vi "Global Log Handling Capability Example.vi"() -> ()   [LabVIEW 2017, in "Global Log Handling Capability Example.lvlib"]
doc: "### Global Log Handling Capability(Global Log Handling Capability Example.vi)\n\n#### Overview\n\nDemonstrates global log handling capability of CSM. This example calls 30 sub-modules that continuously generate events. The main VI captures these events and uses the Global Log APIs to calculate and display key processing metrics, such as LogInQ, changing speed, and handling speed.\n\nUse this example to benchmark global log performance of CSM and as a reference for custom implementations.\n\n#### Introduction\n\nThis example demonstrates global log handling capability of CSM. This example calls 30 sub-modules that continuously generate events. The main VI captures these events and uses the Global Log APIs to calculate and display key processing metrics, such as LogInQ, changing speed, and handling speed.\n\nUse this example to benchmark global log performance of CSM and as a reference for custom implementations.\n\n#### Steps\n\nStep 1: Asynchronously call 30 CSM submodules, each of which will then generate events continuously.\n\nStep 2: Starts the CSM Watchdog thread to ensure that all asynchronously started CSM modules exit properly after the main program exits.\n\nStep 3: Use CSM's built-in global log APIs to capture and calculate some typical logging capability figures.\n\nStep 4: Exit the caller and all the other running CSM modules."
uses:
  Global Log Handling Capability Example.lvlib
  user.lib/_NEVSTOP/Communicable State Machine(CSM)/Utility/_support/Periodic String Filter Level.ctl
  user.lib/_NEVSTOP/Communicable State Machine(CSM)/Utility/Periodic String Filter Setting.ctl
  user.lib/_NEVSTOP/Communicable State Machine(CSM)/Communicable State Machine.lvlib
  user.lib/_NEVSTOP/Communicable State Machine(CSM)/addons/Watchdog/CSM Watchdog.lvlib
  user.lib/_NEVSTOP/Communicable State Machine(CSM)/_Shared/CSM Shared.lvlib
panel:
  out "size(s)":i32
  in  "Module Num":i32=30
  out "log handling Speed(#/s)":dbl(graph)
  out "Since Exiting(s)":dbl format="%.2f"
  out "LogInQ":i32
  out "State History":string
  out "log handling Speed(#/s)":dbl
  out "LogInQ changing Speed(#/s)":dbl
  out "Level":T1
  out "Module Names":string[](array[string])
  in  "Exit Modules":bool
  # "Set before run VI"
  # "#CSM-Example Overview\n\nDemonstrates invoking a CSM submodule in a side loop. Externally, this module interacts like a standard CSM submodule, but note its specific API and status change behavior."
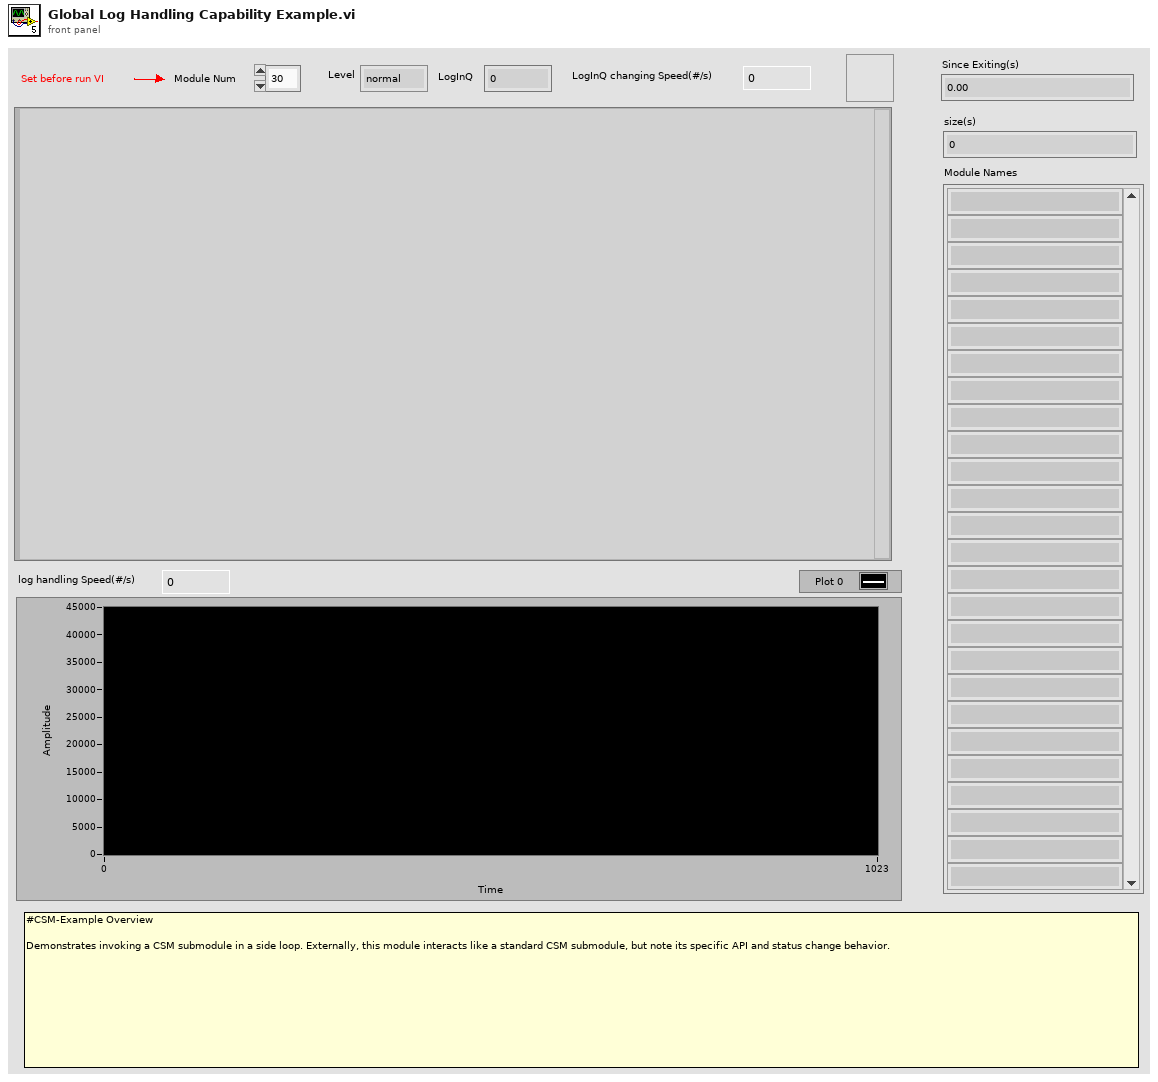
[diagram p1: front panel]
types:
  T1 = typedef "Communicable State Machine.lvlib/Periodic String Filter Level.ctl" = enum16{"normal", "L1", "L2", "L3", "L4"}
  T2 = typedef "Communicable State Machine.lvlib/Periodic String Filter Setting.ctl" = cluster{"threashold(#/s)":dbl, "Check Peroid(s)":dbl}
  T3 = typedef "Communicable State Machine.lvlib/_CSM_GlobalLog_MSG.ctl" = cluster{"Name (\"\" to Use UUID)":string, "Current State":string, "Arguments":string, "Source Message":T4, "Source Module":string, "Complete(T)/Start(F)":bool, "LogType":T5, "Time Stamp":timestamp}
  T4 = typedef "Communicable State Machine.lvlib/_CSM_Response Source Message.ctl" = cluster{"‘State":string, "’Arguments":string, "’Error":errorcluster}
  T5 = typedef "Communicable State Machine.lvlib/_CSM_GlobalLog_MSG_TYPE.ctl" = enum16{"User Log", "State Change", "Status", "Interrupt", "Register", "Unregister", "Error Log", "Module Created", "Module Destroyed"}
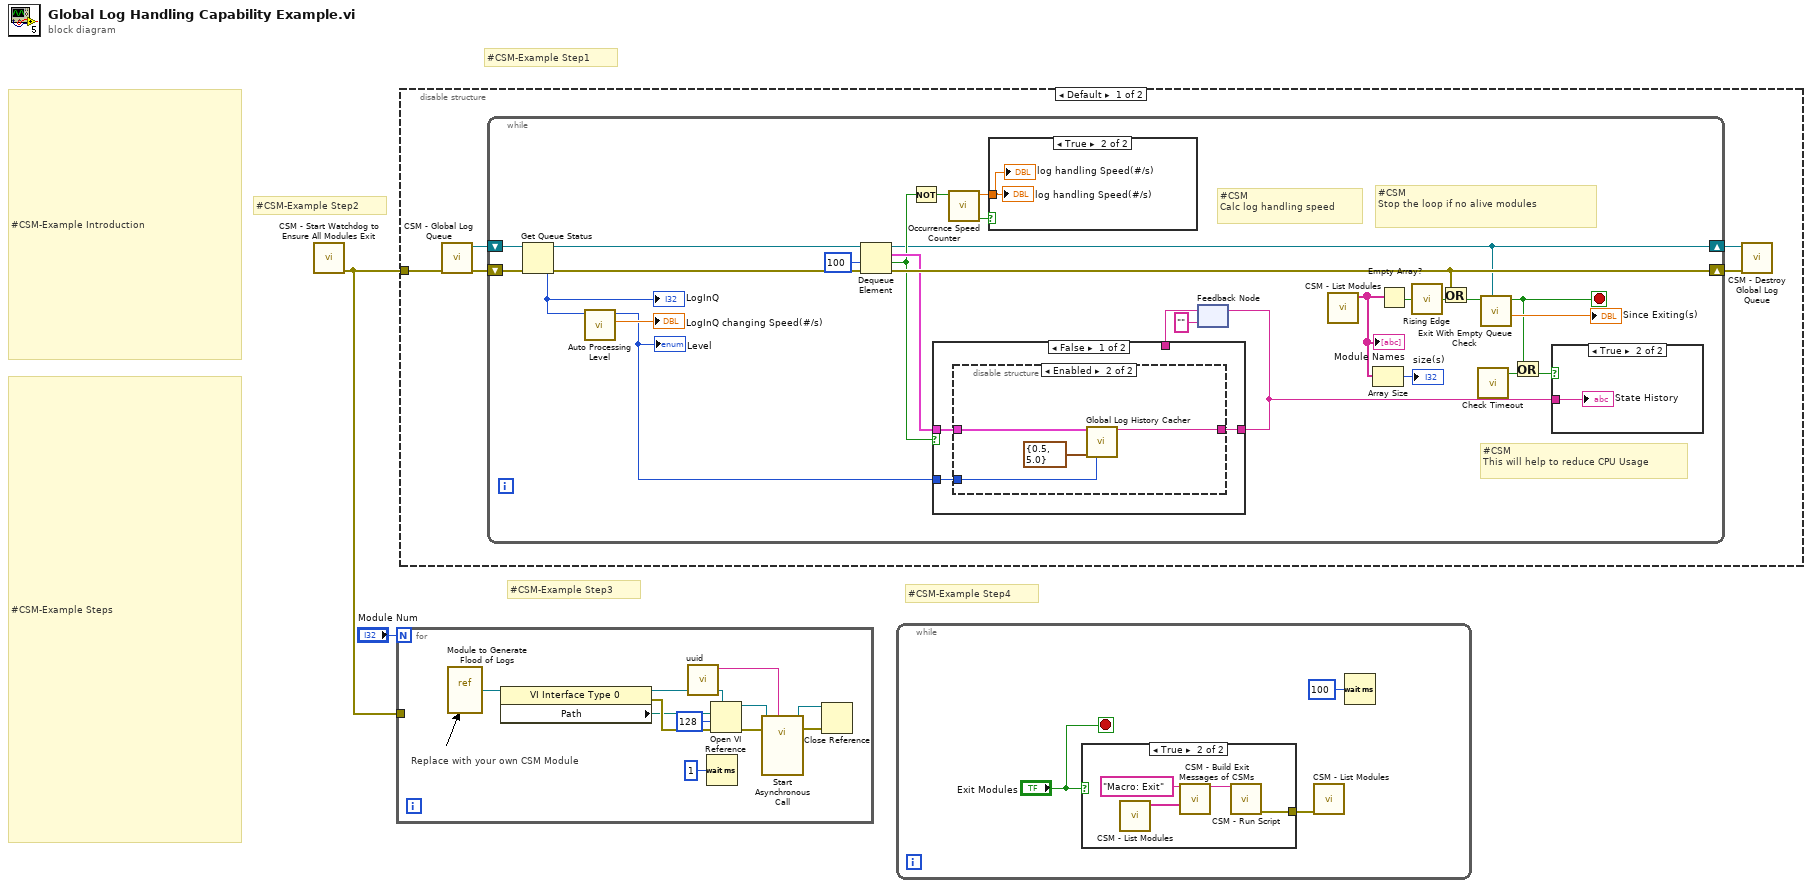
[diagram p0: block diagram]
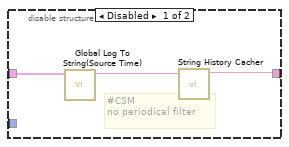
[diagram p3: hidden frame]
diagram:
  # "#CSM-Example Step4"
  # "#CSM-Example Step3"
  # "#CSM-Example Step2"
  # "#CSM-Example Step1"
  # "#CSM-Example Steps"
  # "#CSM-Example Introduction"
  n1 = call "CSM - Start Watchdog to Ensure All Modules Exit.vi"() -> ("error out"=w1:errorcluster)  [unwired: 11 in]
  n2 = for {
    N: "Module Num" -> [_]
    tunnel: w1 -> [_]
    # "Replace with your own CSM Module"
    n3 = vi-ref "Module to Generate Flood of Logs.vi"() -> (w6:refnum<vi>)
    n4 = property class="VI Interface Type 0"(reference=w6) -> (reference out=w10:refnum<vi>, error out=w8:errorcluster, "Path"=w7:path)  [unwired: 1 in]
    n5 = call "uuid.vi"() -> ("UUID"=w4:string)  [unwired: 11 in]
    n6 = Wait (ms)(milliseconds to wait=u32 1) -> ()  [unwired: 1 out]
    n7 = Open VI Reference(type specifier VI Refnum (for type only)=w10, vi path=w7, options=128, error in (no error)=w8) -> (vi reference=w9:refnum<vi>, error out=w5:errorcluster)  [unwired: 2 in]
    n8 = call-by-ref "Start Asynchronous Call"(reference=w9, error in=w5, "Name(\"\" to use uuid)"=w4) -> (reference out=w12:refnum<vi>, error out=w11:errorcluster)  [unwired: 11 in]
    n9 = Close Reference(reference=w12, error in (no error)=w11) -> ()  [unwired: 1 out]
  }
  n10 = disable-structure shown="Default" {
    disable-tunnel: w1 -> [w14 _]
    frame condition #0 (active) {
      n11 = call "CSM - Global Log Queue.vi"("Error In"=w14) -> ("error out"=w17:errorcluster, "GlobalEvent Queue"=w15:refnum<queue>)  [unwired: 9 in]
      n12 = while {
        shift-right: [w44] -> w18
        shift-left: w17 -> [w41]
        shift-right: [w32] -> w16
        shift-left: w15 -> [w45]
        stop <- w25 stop-if-true
        # "#CSM\nCalc log handling speed"
        # "#CSM\nStop the loop if no alive modules"
        # "#CSM\nThis will help to reduce CPU Usage"
        n13 = Get Queue Status(queue=w45, error in (no error)=w41) -> (queue out=w43:refnum<queue>, error out=w42:errorcluster, # elements in queue=w28:i32)  [unwired: 1 in, 5 out]
        "LogInQ" <- w28
        n14 = call "Auto Processing Level.vi"("#Left In Q"=w28) -> ("LogInQ Changing Speed (#/s)"=→"LogInQ changing Speed(#/s)":dbl, "Level"=w27:T1)  [unwired: 8 in, 1 out]
        "Level" <- w27
        n15 = Dequeue Element(queue=w43, timeout in ms (-1)=100, error in (no error)=w42) -> (queue out=w32:refnum<queue>, element=w40:T3, timed out?=w34:bool, error out=w44:errorcluster)
        n16 = Not(x=w34) -> (.not. x?=w33:bool)
        n17 = call "Occurrence Speed Counter.vi"("Occured? (T)"=w33) -> ("New?"=w23:bool, "Speed (#/s)"=w24:dbl)  [unwired: 8 in, 1 out]
        n18 = case shown="True" w23 {
          tunnel: w24 -> [_ w46]
          frame False {
          }
          frame True {
            "log handling Speed(#/s)" <- w46
            "log handling Speed(#/s)" <- w46
          }
        }
        n19 = feedback #1("" ("String Cache")) -> (w36:string)
        n20 = case shown="False" w34 {
          tunnel: w40 -> [w49 _]
          tunnel: [w48 w57] -> w37
          tunnel: w36 -> [_ w57]
          tunnel: w27 -> [w47 _]
          frame False {
            n21 = disable-structure shown="Enabled" {
              disable-tunnel: w49 -> [w52 w55]
              disable-tunnel: [w50 w56] -> w48
              disable-tunnel: w47 -> [_ w54]
              frame Disabled {
                # "#CSM \nno periodical filter"
                n22 = call "Global Log To String(Source Time).vi"("Log"=w52) -> ("Log String"=w51:string)  [unwired: 9 in]
                n23 = call "String History Cacher.vi"("String"=w51) -> ("String Cache"=w50:string)  [unwired: 10 in]
              }
              frame Enabled {
                n24 = call "Global Log History Cacher.vi"("Cross CSM Data"=w55, "Settings"=T2 {"threashold(#/s)"=0.5, "Check Peroid(s)"=5.0}, "Level (Normal)"=w54) -> ("String Cache"=w56:string)  [unwired: 12 in]
              }
            }
          }
          frame True {
          }
        }
        n25 = feedback-in #1(w37) -> ()
        n26 = call "CSM - List Modules.vi"() -> ("Module Names"=w20:string[])  [unwired: 10 in, 1 out]
        "Module Names" <- w20
        n27 = Array Size(array=w20) -> (size(s)=→"size(s)":i32)
        n28 = Empty Array?(array=w20) -> (empty?=w22:bool)
        n29 = call "Rising Edge.vi"("Signal"=w22) -> ("Rising Edge"=w21:bool)
        n30 = Or(x=w44, y=w21) -> (x .or. y?=w30:bool)
        n31 = call "Check Timeout.vi"() -> ("Timeout"=w38:bool)  [unwired: 8 in]
        n32 = call "Exit With Empty Queue Check.vi"("Queue"=w32, "Stop"=w30) -> ("Since Exiting (S)"=→"Since Exiting(s)":dbl, "Exit"=w25:bool)  [unwired: 8 in]
        n33 = Or(x=w25, y=w38) -> (x .or. y?=w31:bool)
        n34 = case shown="True" w31 {
          tunnel: w37 -> [_ w58]
          frame False {
          }
          frame True {
            "State History" <- w58
          }
        }
      }
      n35 = call "CSM - Destroy Global Log Queue.vi"("Error In"=w18, "Global Log Queue"=w16) -> ()  [unwired: 9 in, 1 out]
    }
    frame condition #1 {
    }
  }
  n36 = while {
    stop <- "Exit Modules" stop-if-true
    n37 = case shown="True" "Exit Modules" {
      tunnel: [_ w63] -> w60
      frame False {
      }
      frame True {
        n38 = call "CSM - List Modules.vi"() -> ("Module Names"=w65:string[])  [unwired: 10 in, 1 out]
        n39 = call "CSM - Build Exit Messages of CSMs.vi"("State With Arguments (\"Macro: Exit“)"="Macro: Exit" ("State with Arguments(\"Macro: Exit“)"), "CSMs"=w65) -> ("States"=w62:string)  [unwired: 13 in]
        n40 = call "CSM - Run Script.vi"("CSM Scripts"=w62) -> ("error out"=w63:errorcluster)  [unwired: 12 in, 2 out]
      }
    }
    n41 = call "CSM - List Modules.vi"("Error In"=w60) -> ()  [unwired: 9 in, 2 out]
    n42 = Wait (ms)(milliseconds to wait=u32 100) -> ()  [unwired: 1 out]
  }
